vi "subGetLibraryDependencies.vi"(8 "error in (no error)":errorcluster, 9 "Source dist":map{string, set{string}}(c390), 11 "Project ref":refnum<vi>) -> (0 "error out":errorcluster, 1 "Library refs":map{string, refnum<vi>}(c390), 3 "Deps":map{string, set{string}}(c390))   [LabVIEW 2020, in "SolutionBuilder.lvlib" / "SolutionBuilder.lvclass"]
uses:
  SolutionBuilder.lvclass
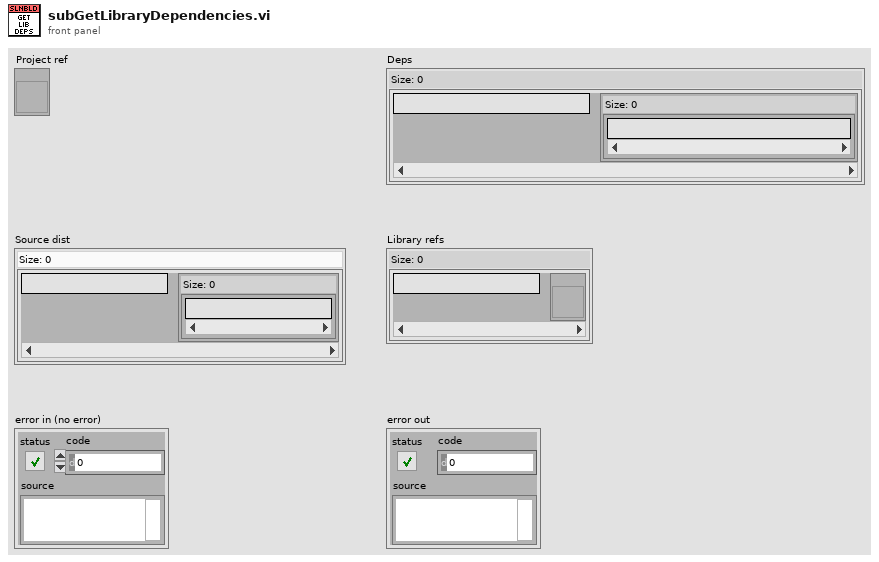
[diagram p1: front panel]
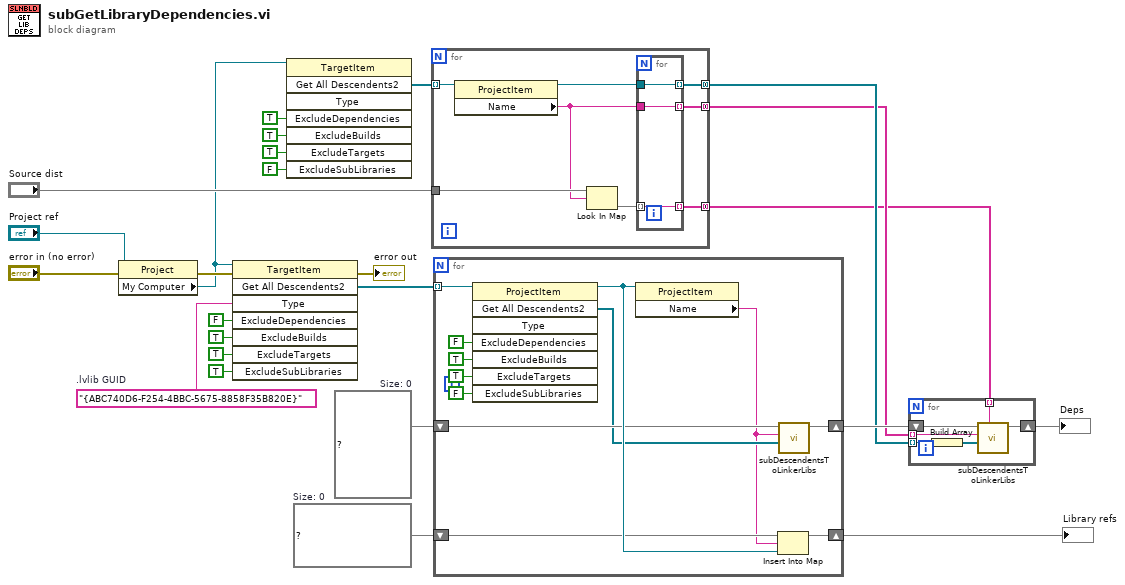
[diagram p0: block diagram]
diagram:
  w16 = map{string, refnum<vi>} {}  # Size: 0
  w24 = map{string, set{string}} {}  # Size: 0
  w14 = "{ABC740D6-F254-4BBC-5675-8858F35B820E}"  # .lvlib GUID
  n1 = property class="Project"(reference="Project ref", error in="error in (no error)") -> (error out=w25:errorcluster, "My Computer"=w1:refnum<vi>)  [unwired: 1 out]
  n2 = invoke class="TargetItem" method="Get All Descendents2"(reference=w1, error in=w25, "Type"=w14, "ExcludeDependencies"=FALSE, "ExcludeBuilds"=TRUE, "ExcludeTargets"=TRUE, "ExcludeSubLibraries"=TRUE) -> (error out=→"error out":errorcluster, "Get All Descendents2"=w7:refnum<vi>[])  [unwired: 1 in, 6 out]
  n3 = invoke class="TargetItem" method="Get All Descendents2"(reference=w1, "ExcludeDependencies"=TRUE, "ExcludeBuilds"=TRUE, "ExcludeTargets"=TRUE, "ExcludeSubLibraries"=FALSE) -> ("Get All Descendents2"=w13:refnum<vi>[])  [unwired: 3 in, 7 out]
  n4 = for {
    tunnel: w13 -> [w33] mode=indexing
    tunnel: "Source dist" -> [w32]
    tunnel: [w28] -> w4 mode=concatenating
    tunnel: [w27] -> w3 mode=concatenating
    tunnel: [w26] -> w2 mode=concatenating
    n5 = property class="ProjectItem"(reference=w33) -> (reference out=w29:refnum<vi>, "Name"=w30:string)  [unwired: 1 in, 1 out]
    n6 = Look In Map(map=w32, key=w30) -> (value=w31:set{string})  [unwired: 1 in, 1 out]
    n7 = for {
      tunnel: w31 -> [w36] mode=indexing
      tunnel: [w36] -> w26 mode=indexing
      tunnel: [w35] -> w27 mode=indexing
      tunnel: w30 -> [w35]
      tunnel: [w34] -> w28 mode=indexing
      tunnel: w29 -> [w34]
    }
  }
  n8 = for {
    tunnel: w7 -> [w47] mode=indexing
    shift-right: [w48] -> w6
    shift-left: w24 -> [w39]
    shift-right: [w41] -> w15
    shift-left: w16 -> [w40]
    n9 = invoke class="ProjectItem" method="Get All Descendents2"(reference=w47, "ExcludeDependencies"=FALSE, "ExcludeBuilds"=TRUE, "ExcludeTargets"=TRUE, "ExcludeSubLibraries"=FALSE) -> (reference out=w42:refnum<vi>, "Get All Descendents2"=w38:refnum<vi>[])  [unwired: 3 in, 6 out]
    n10 = property class="ProjectItem"(reference=w42) -> ("Name"=w37:string)  [unwired: 1 in, 2 out]
    n11 = Insert Into Map(map in=w40, key=w37, value=w42) -> (map out=w41:map{string, refnum<vi>})  [unwired: 2 out]
    n12 = call "subDescendentsToLinkerLibs.vi"("All descendents"=w38, "Name"=w37, "Map in"=w39) -> ("Map out"=w48:map{string, set{string}})  [unwired: 8 in]
  }
  "Library refs" <- w15
  n13 = for {
    tunnel: w4 -> [w52] mode=indexing
    tunnel: w3 -> [w51] mode=indexing
    tunnel: w2 -> [w50] mode=indexing
    shift-right: [w53] -> w5
    shift-left: w6 -> [w54]
    n14 = Build Array(w52) -> (w49:refnum<vi>[])
    n15 = call "subDescendentsToLinkerLibs.vi"("Build spec override"=w50, "All descendents"=w49, "Name"=w51, "Map in"=w54) -> ("Map out"=w53:map{string, set{string}})  [unwired: 7 in]
  }
  "Deps" <- w5
